vi "Check Valid UI Selection.vi"(8 "error in (no error)":errorcluster, 10 "valid":bool, 11 "Operator UI in":refnum<class "Controller UI.lvclass">) -> (0 "error out":errorcluster, 3 "Operator UI out":refnum<class "Controller UI.lvclass">)   [LabVIEW 2016, in "Controller UI.lvlib" / "Controller UI.lvclass"]
uses:
  <userlib>/Common Components/Controller UI/Controller UI.lvclass
  <userlib>/Common Components/Controller UI/Controller UI.lvclass/Controller UI.ctl
  <userlib>/Common Components/Controller UI/Accessors/Read Run.vi
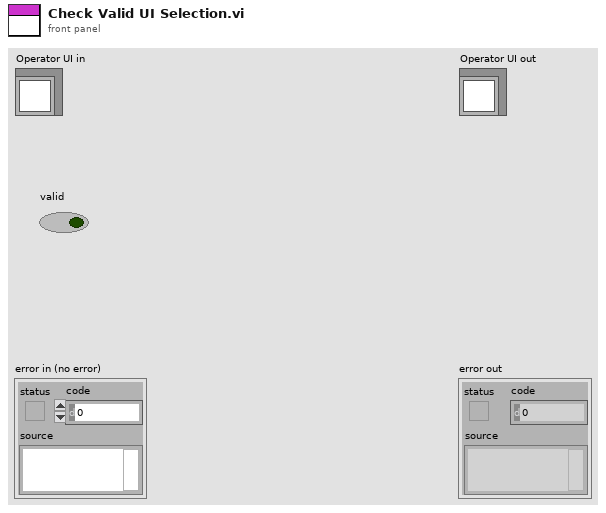
[diagram p1: front panel]
types:
  T1 = enum8{"Enabled", "Disabled", "Disabled and Grayed Out"}
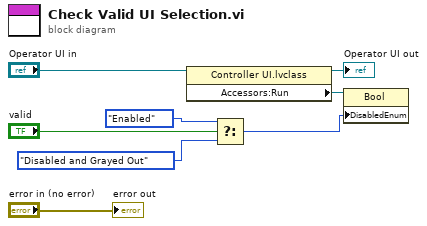
[diagram p0: block diagram]
diagram:
  n1 = property class="Controller UI.lvclass"(reference="Operator UI in") -> (reference out=→"Operator UI out":refnum<class "Controller UI.lvclass">, "Accessors:Run"=w2:refnum<vi>)  [unwired: 1 in, 1 out]
  n2 = Select(t=T1."Enabled" ("Disabled"), s="valid", f=T1."Disabled and Grayed Out" ("Disabled")) -> (s? t:f=w6:T1)
  n3 = property class="Bool"(reference=w2, "DisabledEnum"=w6) -> ()  [unwired: 1 in, 2 out]
  "error out" <- "error in (no error)"
